vi "SetNumbersAndOperationMethod - Reentrant.vi"(6 "error in (no error)":errorcluster, 8 "Operator":enum16{"Add", "Divide", "Multiple", "Subtract"}(ring), 9 "Numeric 2":dbl, 10 "Numeric":dbl, 11 "SimpleArithmetic in":refnum<class "SimpleArithmetic - Reentrant.lvclass">) -> (0 "error out":errorcluster, 3 "SimpleArithmetic out":refnum<class "SimpleArithmetic - Reentrant.lvclass">)   [LabVIEW 2013, in "SimpleArithmetic - Reentrant.lvclass"]
uses:
  SimpleArithmetic - Reentrant.lvclass
  SimpleArithmetic - Reentrant.lvclass/SimpleArithmetic - Reentrant.ctl
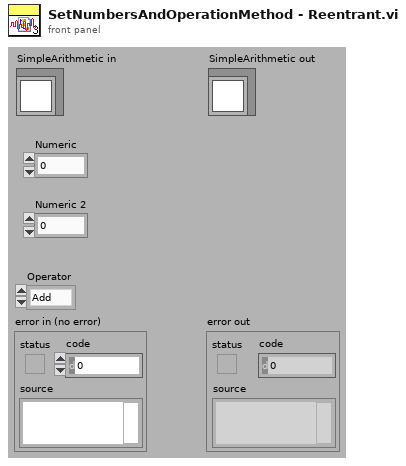
[diagram p1: front panel]
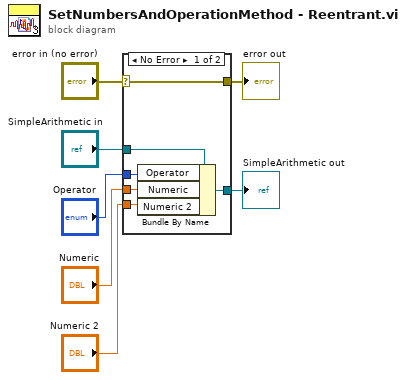
[diagram p0: block diagram]
diagram:
  n1 = case shown="No Error" "error in (no error)" {
    selector: "error in (no error)" -> [w13 w15]
    tunnel: [w13 w15] -> w6
    tunnel: [w11 w14] -> w4
    tunnel: "SimpleArithmetic in" -> [w12 w14]
    tunnel: "Operator" -> [w10 _]
    tunnel: "Numeric" -> [w9 _]
    tunnel: "Numeric 2" -> [w8 _]
    frame No Error {
      n2 = Bundle By Name(cluster=w12, "Operator"=w10, "Numeric"=w9, "Numeric 2"=w8) -> (w11:refnum<class "SimpleArithmetic - Reentrant.lvclass">)
    }
    frame Error {
    }
  }
  "error out" <- w6
  "SimpleArithmetic out" <- w4
